vi "Format Item Names.vi"(7 "Displayed Indices":i32[](array[numeric]), 8 "Flat View?":bool, 9 "Abbreviate Names?":bool, 11 "New Item Data":refnum<class "Item.lvclass">[](array[class])) -> (1 "Number of Items Added":i32, 3 "Formatted VI Data to Display":refnum<class "Item.lvclass">[](array[class]))   [LabVIEW 2020, in "VI Properties Editor.lvlib"]
doc: "Formats the item names to be displayed, based on <B>Abbreviate Names?</B>, <B>Flat View</B>, and if modifications have been made."
uses:
  VI Properties Editor.lvlib
  Classes/Item/Item.lvclass
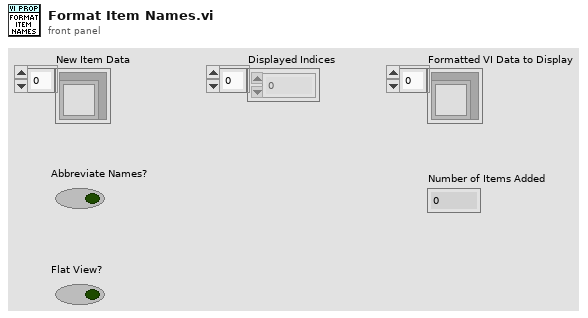
[diagram p1: front panel]
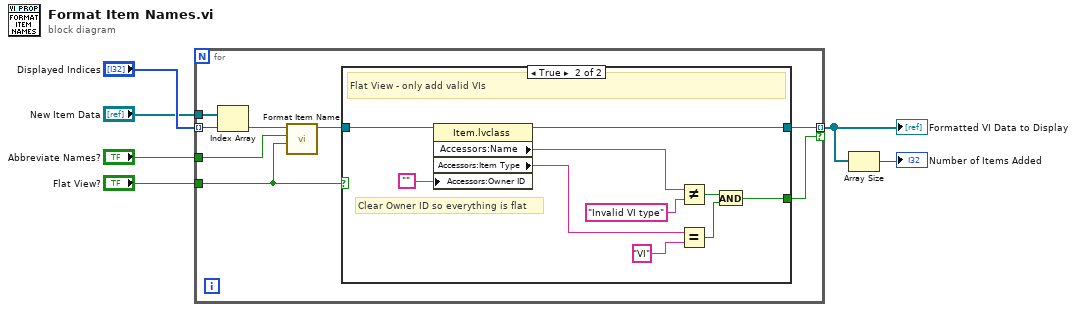
[diagram p0: block diagram]
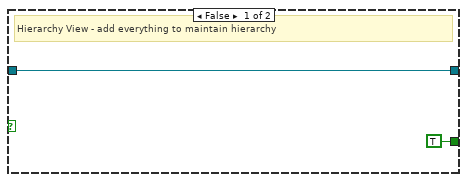
[diagram p2: hidden frame]
diagram:
  n1 = for {
    tunnel: "New Item Data" -> [w14]
    tunnel: "Displayed Indices" -> [w13] mode=indexing
    tunnel: [w9] -> w1 mode=indexing if=w8
    tunnel: "Abbreviate Names?" -> [w11]
    tunnel: "Flat View?" -> [w7]
    n2 = Index Array(array=w14, index=w13) -> (element=w12:refnum<class "Item.lvclass">)
    n3 = call-dynamic "Format Item Name.vi"("Flat View?"=w7, "Abbreviate Names?"=w11, "Item in"=w12) -> ("Item out"=w10:refnum<class "Item.lvclass">)  [unwired: 7 in, 1 out]
    n4 = case shown="True" w7 {
      tunnel: w10 -> [w16 w19]
      tunnel: [w16 w18] -> w9
      tunnel: [TRUE w17] -> w8
      frame False {
        # "Hierarchy View - add everything to maintain hierarchy"
      }
      frame True {
        # "Clear Owner ID so everything is flat"
        # "Flat View - only add valid VIs"
        n5 = property class="Item.lvclass"(reference=w19, "Accessors:Owner ID"="") -> (reference out=w18:refnum<class "Item.lvclass">, "Accessors:Name"=w20:string, "Accessors:Item Type"=w22:string)  [unwired: 1 in, 1 out]
        n6 = Not Equal?(x=w20, y="Invalid VI type") -> (x != y?=w24:bool)
        n7 = Equal?(x=w22, y="VI") -> (x = y?=w25:bool)
        n8 = And(x=w24, y=w25) -> (x .and. y?=w17:bool)
      }
    }
  }
  "Formatted VI Data to Display" <- w1
  n9 = Array Size(array=w1) -> (size(s)=→"Number of Items Added":i32)
